vi "PicoScope2000aExampleRapidBlockBulkMSO.vi"() -> ()   [LabVIEW 2009]
uses:
  <vilib>/Waveform/DWDTOps.llb/DWDT Analog to Digital.vi
panel:
  in  "Port 0 Settings":cluster{"Enabled":bool, "Logic Level":i16} {"Logic Level" items=["1.5V TTL", "2.5V CMOS"]}
  out "Port 0 Digital Waveform Graph":digitalwaveform(graph)
  in  "Rapid Block Acquisition Settings":T1 {"Down Sample Ratio" min=1 step=1; "Down-Sample Mode" items=["None", "Aggregate", "Decimate", "Average"]}
  in  "Channel A Settings":T2 {"Range" items=["20 mV", "50 mV", "100 mV", "200 mV", "500 mV", "1 V", "2 V", "5 V", "10 V", "20 V"]; "Coupling" items=["AC", "DC"]}
  out "Properties Panel":T3 {"Max Total Capture Time Available (sec)" format="%.3p"; "Sample Frequency" format="%.3p"; "Sample Internal" format="%.3p"; "Max Samples Available" format="%.3p"; "Total Capture Time (sec)" format="%.3p"}
  in  "Trigger Settings":T4 {"Trigger Direction" items=["Rising", "Falling"]}
  out "Capture Complete":bool
  in  "Run":bool
  out "Channel A":T5(graph)
  in  "Capture Index":u32
  in  "stop":bool
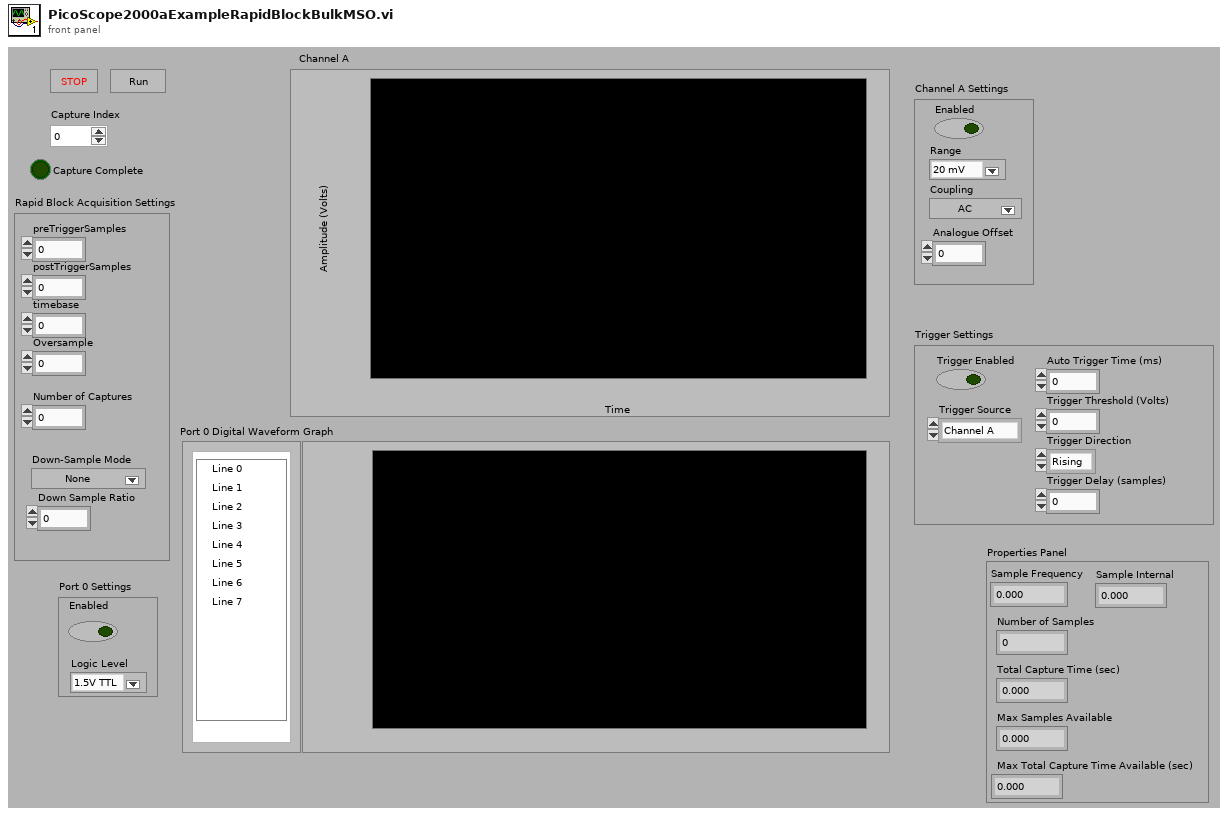
[diagram p1: front panel]
types:
  T1 = cluster{"preTriggerSamples":u32, "postTriggerSamples":u32, "timebase":u32, "Down-Sample Mode":i32, "Down Sample Ratio":u32, "Oversample":i16, "Number of Captures":u32}
  T2 = cluster{"Enabled":bool, "Coupling":i16, "Range":u16, "Analogue Offset":sgl}
  T3 = cluster{"Sample Frequency":sgl, "Sample Internal":sgl, "Max Samples Available":i32, "Number of Samples":u32, "Total Capture Time (sec) ":sgl, "Max Total Capture Time Available (sec)":sgl}
  T4 = cluster{"Trigger Enabled":bool, "Trigger Source":enum16{"Channel A", "Channel B", "Channel C", "Channel D", "Ext."}, "Trigger Threshold (Volts)":dbl, "Trigger Direction":u16, "Trigger Delay (samples)":u32, "Auto Trigger Time (ms)":i16}
  T5 = cluster{i32, "Sample Internal":sgl, "Data (Volts)":dbl[]}
  T6 = cluster{"Driver Version":string, "USB Version":string, "Hardware":string, "Variant":string, "Batch and Serial":string, "Cal Date":string, "Kernel Version":string, "Digital HW Version":string, "Analogue HW Version":string, "Firmware 1":string, "Firmware 2":string, "MSO":bool, "Number of Channels":i16}
  T7 = cluster{"preTriggerSamples":u32, "postTriggerSamples":u32, "timebase":u32, "Oversample":i16, "Down-Sample Mode":i32, "Down Sample Ratio":u32}
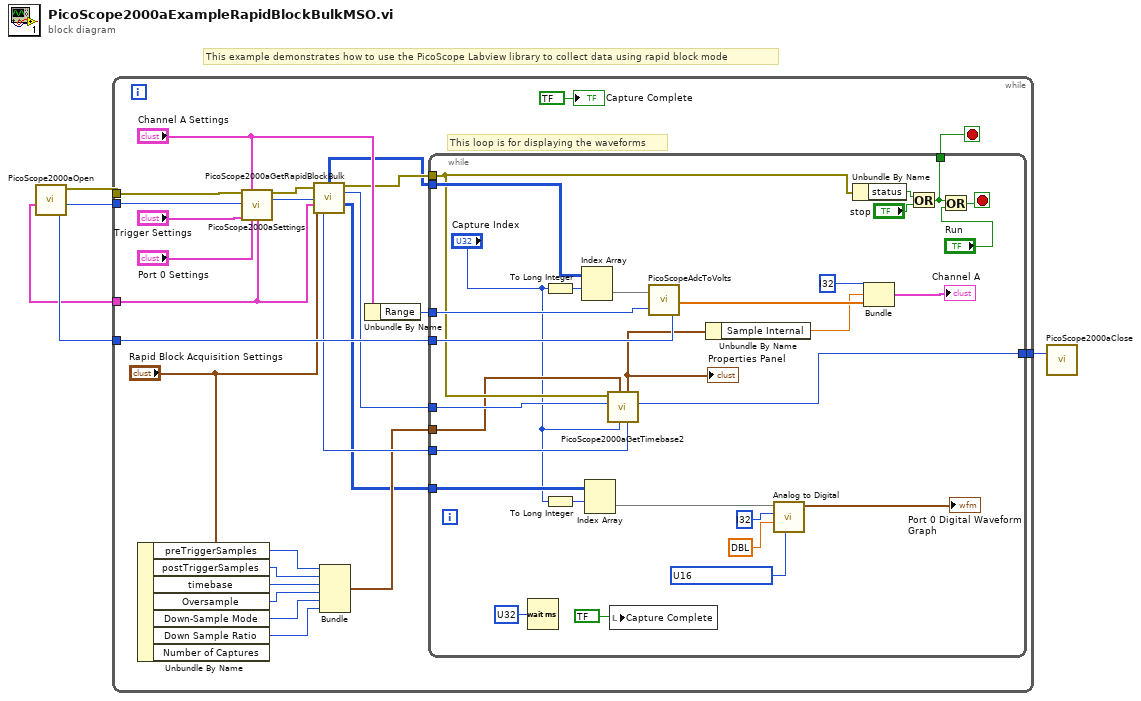
[diagram p0: block diagram]
diagram:
  # "This example demonstrates how to use the PicoScope Labview library to collect data using rapid block mode"
  n1 = call "PicoScope2000aOpen.vi"() -> ("Max Adc value"=w3:i16, "handle"=w4:i16, "error out"=w5:errorcluster, "Device Info"=w1:T6)  [unwired: 4 in]
  n2 = while {
    tunnel: w4 -> [w28]
    tunnel: w5 -> [w29]
    tunnel: w3 -> [w27]
    tunnel: [w24] -> w2
    tunnel: w1 -> [w17]
    stop <- w31 stop-if-true
    # "This loop is for displaying the waveforms"
    n3 = Unbundle By Name("Rapid Block Acquisition Settings") -> ("preTriggerSamples"=w15:u32, "postTriggerSamples"=w14:u32, "timebase"=w13:u32, "Oversample"=w12:i16, "Down-Sample Mode"=w11:i32, "Down Sample Ratio"=w8:u32)  [unwired: 1 out]
    n4 = call "PicoScope2000aSettings.vi"("error in"=w29, "Channel A Settings"="Channel A Settings", "handle in"=w28, "Trigger Settings"="Trigger Settings", "Port 0 Settings"="Port 0 Settings", "Device Info"=w17) -> ("error out"=w20:errorcluster, "handle out"=w22:i16)  [unwired: 7 in, 1 out]
    n5 = call "PicoScope2000aGetRapidBlockBulk.vi"("error in"=w20, "handle in"=w22, "Device Info"=w17, "Rapid Block Acquisition Settings"="Rapid Block Acquisition Settings") -> ("Channel A Buffer"=w19:i16[][], "error out"=w21:errorcluster, "handle out"=w18:i16, "Port 0 Buffer"=w7:i16[][], "Num samples"=w16:u32)  [unwired: 3 in, 4 out]
    n6 = Bundle("preTriggerSamples"=w15, "postTriggerSamples"=w14, "timebase"=w13, "Oversample"=w12, "Down-Sample Mode"=w11, "Down Sample Ratio"=w8) -> (w10:T7)  [unwired: 1 in]
    n7 = Unbundle By Name("Channel A Settings") -> ("Range"=w26:u16)
    n8 = while {
      tunnel: [w60] -> w31
      tunnel: w19 -> [w54]
      tunnel: w21 -> [w50]
      tunnel: w27 -> [w53]
      tunnel: w26 -> [w51]
      tunnel: w18 -> [w49]
      tunnel: [w48] -> w24
      tunnel: w16 -> [w47]
      tunnel: w10 -> [w46]
      tunnel: w7 -> [w37]
      stop <- w59 stop-if-true
      w39 = u16 ? items=["unsigned binary", "offset binary", "2's complement"] ("data format (offset binary)")
      n9 = Wait (ms)(milliseconds to wait=u32 ?) -> ()  [unwired: 1 out]
      n10 = To Long Integer(number="Capture Index") -> (32bit integer=w33:i32)
      n11 = To Long Integer(number="Capture Index") -> (32bit integer=w34:i32)
      n12 = Index Array(array=w54, index (row)=w33) -> (element=w52:i16[])  [unwired: 1 in]
      n13 = Index Array(array=w37, index (row)=w34) -> (element=w38:i16[])  [unwired: 1 in]
      n14 = call "PicoScope2000aGetTimebase2.vi"("Number of Samples"=w47, "Memory Segment"="Capture Index", "Acquisition Settings"=w46, "handle in"=w49, "error in (no error)"=w50) -> ("handle out"=w48:i16, "Properties Panel"=w42:T3)  [unwired: 4 in, 1 out]
      "Properties Panel" <- w42
      n15 = local write "Capture Complete"(bool ? ("Capture Complete")) -> ()
      n16 = call "PicoScopeAdcToVolts.vi"("Max_adc"=w53, "Range Index"=w51, "Data"=w52) -> ("Data (Volts)"=w44:dbl[])
      n17 = Unbundle By Name(w42) -> ("Sample Internal"=w36:sgl)
      n18 = call-poly <vilib>:"Analog to Digital.vi"("data format (offset binary)"=w39, "full-scale range (pk-pk)"=dbl ?, "resolution (16 bit)"=i32 ?, "analog waveform"=w38) -> ("digital waveform"=→"Port 0 Digital Waveform Graph":digitalwaveform)  [unwired: 4 in, 3 out]
      n19 = Unbundle By Name(w50) -> ("status"=w55:bool)
      n20 = Bundle(i32 ?, "Sample Internal"=w36, "Data (Volts)"=w44) -> (→"Channel A":T5)  [unwired: 1 in]
      n21 = Or(x=w55, y="stop") -> (x .or. y?=w60:bool)
      n22 = Or(x=w60, y="Run") -> (x .or. y?=w59:bool)
    }
    "Capture Complete" <- bool ? ("Capture Complete")
  }
  n23 = call "PicoScope2000aClose.vi"("handle"=w2) -> ()
